vi "DiffDriveOdom_RelativeTrajectory_EXECUTE.vi"(5 "Track Width FT":dbl, 7 "Max Speed\nFT/SEC":dbl, 8 "Init":bool, 9 "Gyro Continous\n (inc counterclockwise)\nDEG":dbl, 10 "Right Distance FT":dbl, 11 "Left Distance FT":dbl) -> (0 "AtReference":bool, 1 "Right Speed Target":dbl, 2 "Left Speed Target":dbl, 4 "Odometry Pose Meters":T1={"TRANSLATION"={"X"=0.0, "Y"=0.0}, "ROTATION"={"VALUE"=0.0, "COS"=1.0, "SIN"=0.0}} {"ROTATION"."SIN" format="%13.4f"; "ROTATION"."COS" format="%13.4f"; "ROTATION"."VALUE" format="%13.4f"; "TRANSLATION"."Y" format="%14.3f"; "TRANSLATION"."X" format="%14.3f"})   [LabVIEW 2019]
uses:
  <vilib>/Rock Robotics/WPI/ThirdParty/JAS_Junk/TrajLib/Trajectory_Library.lvlib
  DiffDriveOdom_Trajectory_Globals.vi
  <vilib>/Rock Robotics/WPI/ThirdParty/JAS_Junk/TrajLib/TypeDef/TRANSLATION2D.ctl
  <vilib>/Rock Robotics/WPI/ThirdParty/JAS_Junk/TrajLib/TypeDef/ROTATION2D.ctl
  <vilib>/Rock Robotics/WPI/ThirdParty/JAS_Junk/TrajLib/TypeDef/POSE2D.ctl
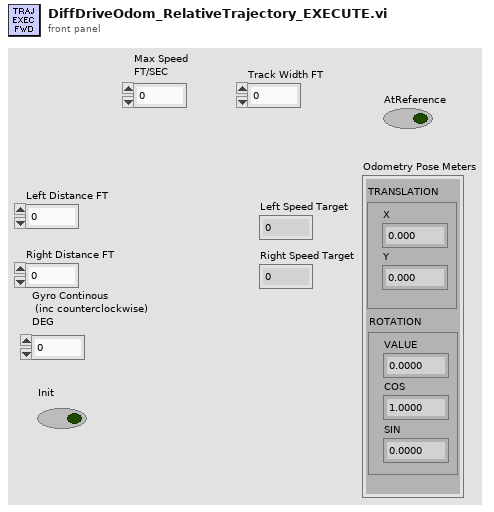
[diagram p1: front panel]
types:
  T1 = typedef "Trajectory_Library.lvlib/POSE2D.ctl" = cluster{"TRANSLATION":T2, "ROTATION":T3}
  T2 = typedef "Trajectory_Library.lvlib/TRANSLATION2D.ctl" = cluster{"X":dbl, "Y":dbl}
  T3 = typedef "Trajectory_Library.lvlib/ROTATION2D.ctl" = cluster{"VALUE":dbl, "COS":dbl, "SIN":dbl}
  T4 = typedef "Trajectory_Library.lvlib/TRAJECTORY.ctl" = cluster{"TotalTImeSecs":dbl, "States":T5[]}
  T5 = typedef "Trajectory_Library.lvlib/TRAJ_STATE.ctl" = cluster{"TimeSeconds":dbl, "Velocity":dbl, "Acceleration":dbl, "POSE":T1, "Curvature":dbl}
  T6 = typedef "Trajectory_Library.lvlib/RAMSETE_EXE_TUNING.ctl" = cluster{"B":dbl, "Zeta":dbl, "X Tolerance M":dbl, "Y Tolerance M":dbl, "Heading Tolerance RAD":dbl, "Track Width M":dbl, "Max Speed M/S":dbl}
  T7 = typedef "Trajectory_Library.lvlib/RAMSETE.ctl" = cluster{"B":dbl, "Zeta":dbl, "poseTolerance":T1, "poseError":T1, "Enabled":bool}
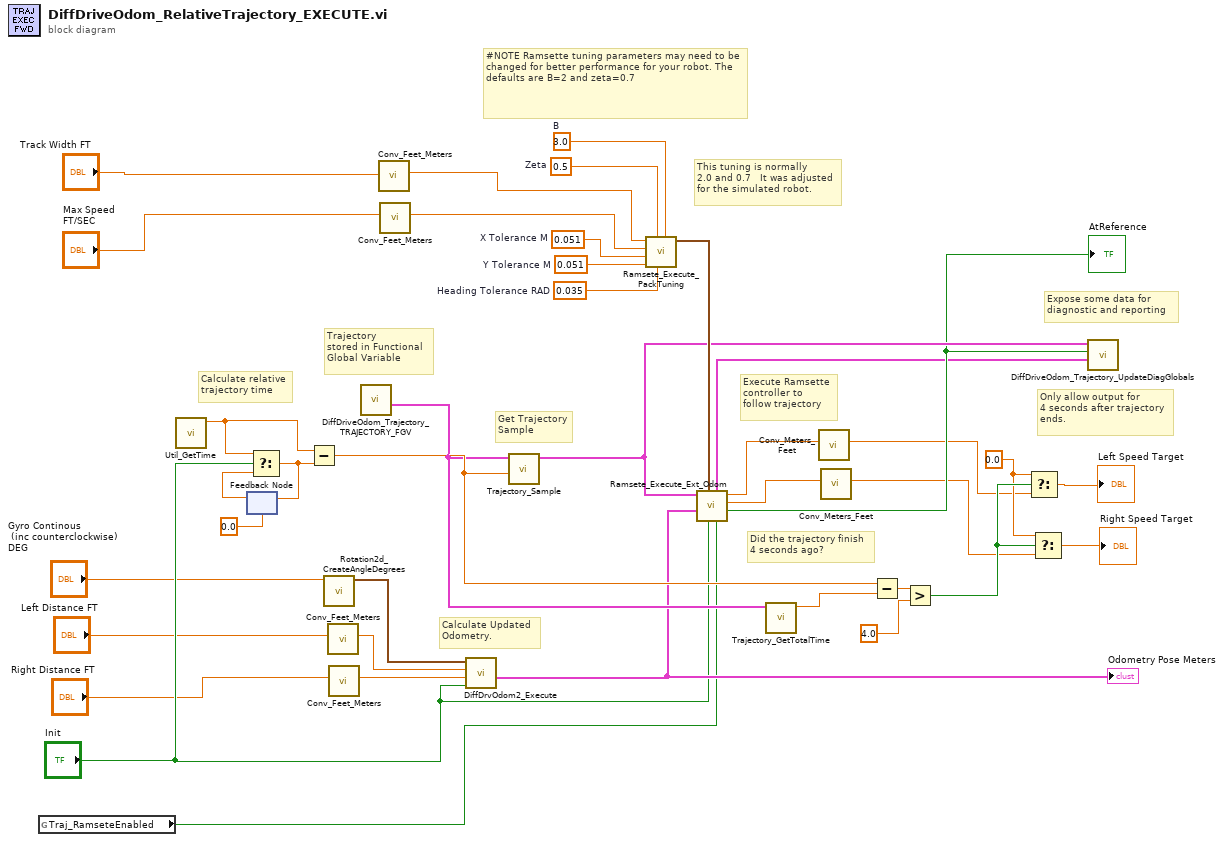
[diagram p0: block diagram]
diagram:
  w26 = 0.051  # X Tolerance M
  w25 = 0.051  # Y Tolerance M
  w24 = 0.5  # Zeta
  w23 = 0.035  # Heading Tolerance RAD
  w22 = 3.0  # B
  w34 = 0.0 ("t")
  # "Execute Ramsette\ncontroller to \nfollow trajectory"
  # "Calculate Updated\nOdometry."
  # "This tuning is normally\n2.0 and 0.7   It was adjusted\nfor the simulated robot."
  # "Expose some data for\ndiagnostic and reporting"
  # "Did the trajectory finish\n4 seconds ago?"
  # "Get Trajectory\nSample"
  # "Trajectory\nstored in Functional\nGlobal Variable"
  # "Calculate relative\ntrajectory time"
  # "#NOTE Ramsette tuning parameters may need to be changed for better performance for your robot. The defaults are B=2 and zeta=0.7"
  # "Only allow output for\n4 seconds after trajectory\nends."
  n1 = global read "DiffDriveOdom_Trajectory_Globals.vi" "Traj_RamseteEnabled"() -> (w12:bool)
  n2 = call <vilib>:"Util_GetTime.vi"() -> ("FPGA_Time_Seconds"=w29:dbl)  [unwired: 9 in, 2 out]
  n3 = feedback #1(0.0 ("TIME")) -> (w30:dbl)
  n4 = Select(t=w29, s="Init", f=w30) -> (s? t:f=w31:dbl)
  n5 = feedback-in #1(w31) -> ()
  n6 = Subtract(x=w29, y=w31) -> (x-y=w38:dbl)
  n7 = call <vilib>:"Rotation2d_CreateAngleDegrees.vi"("Angle_Degrees"="Gyro Continous\n (inc counterclockwise)\nDEG") -> ("ROTATION"=w18:T3)  [unwired: 10 in]
  n8 = call <vilib>:"Conv_Feet_Meters.vi"("Feet"="Left Distance FT") -> ("Meters"=w20:dbl)  [unwired: 10 in]
  n9 = call <vilib>:"Conv_Feet_Meters.vi"("Feet"="Right Distance FT") -> ("Meters"=w19:dbl)  [unwired: 10 in]
  n10 = call "DiffDriveOdom_Trajectory_TRAJECTORY_FGV.vi"() -> ("outTRAJECTORY"=w28:T4)  [unwired: 11 in]
  n11 = call <vilib>:"Conv_Feet_Meters.vi"("Feet"="Track Width FT") -> ("Meters"=w16:dbl)  [unwired: 10 in]
  n12 = call <vilib>:"Conv_Feet_Meters.vi"("Feet"="Max Speed\nFT/SEC") -> ("Meters"=w15:dbl)  [unwired: 10 in]
  n13 = call <vilib>:"DiffDrvOdom2_Execute.vi"("Init / Reset"="Init", "Right Distance M"=w19, "Left Distance M"=w20, "Gyro Reading"=w18) -> ("Pose Meters"=w17:T1)  [unwired: 6 in, 1 out]
  "Odometry Pose Meters" <- w17
  n14 = call <vilib>:"Trajectory_Sample.vi"("Time"=w38, "InputTRAJECTORY"=w28) -> ("OutputTRAJ_STATE"=w7:T5)  [unwired: 9 in]
  n15 = call <vilib>:"Ramsete_Execute_PackTuning.vi"("B"=w22, "Heading Tolerance RAD"=w23, "Zeta"=w24, "Y Tolerance M"=w25, "X Tolerance M"=w26, "Max Speed M/S"=w15, "Track Width M"=w16) -> ("RAMSETE_EXE_TUNING"=w21:T6)  [unwired: 4 in]
  n16 = call <vilib>:"Ramsete_Execute_Ext_Odom.vi"("Enabled"=w12, "Reset"="Init", "RAMSETE_EXE_TUNING SI"=w21, "Current Pose SI"=w17, "TRAJ_STATE SI"=w7) -> ("AtReference"=w6:bool, "Right Speed Dmd M/S"=w3:dbl, "Left Speed Dmd M/S"=w4:dbl, "outRAMSETE"=w5:T7)  [unwired: 3 in]
  "AtReference" <- w6
  n17 = call <vilib>:"Trajectory_GetTotalTime.vi"("TRAJECTORY"=w28) -> ("TotalTime_Sec"=w27:dbl)  [unwired: 10 in]
  n18 = call <vilib>:"Conv_Meters_Feet.vi"("Meters"=w4) -> ("Feet"=w2:dbl)  [unwired: 10 in]
  n19 = call <vilib>:"Conv_Meters_Feet.vi"("Meters"=w3) -> ("Feet"=w1:dbl)  [unwired: 10 in]
  n20 = Subtract(x=w38, y=w27) -> (x-y=w37:dbl)
  n21 = Greater?(x=w37, y=4.0) -> (0:w35:bool)
  n22 = Select(t=w34, s=w35, f=w2) -> (s? t:f=→"Left Speed Target":dbl)
  n23 = Select(t=w34, s=w35, f=w1) -> (s? t:f=→"Right Speed Target":dbl)
  n24 = call "DiffDriveOdom_Trajectory_UpdateDiagGlobals.vi"("outRAMSETE (SI)"=w5, "AtReference"=w6, "OutputTRAJ_STATE (SI)"=w7) -> ()  [unwired: 9 in]
